vi "Overlay.vi"(9 "RefCnt":cluster{dbl, dbl}[](array[cluster]), 11 "Image In":T1) -> (3 "Image Out":T1)   [LabVIEW 2012]
uses:
  <vilib>/vision/Image Controls.llb/IMAQ Image.ctl
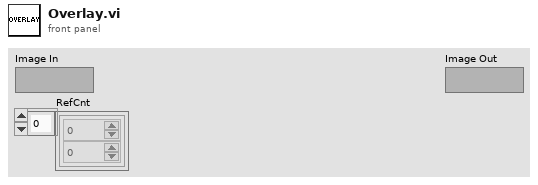
[diagram p1: front panel]
types:
  T1 = typedef "IMAQ Image.ctl" = refnum<image>
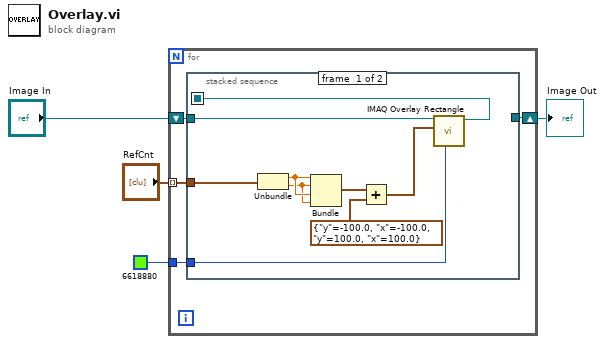
[diagram p0: block diagram]
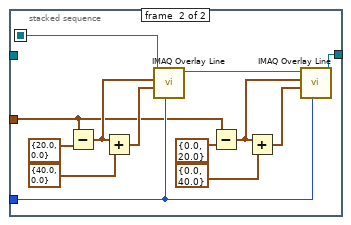
[diagram p2: hidden frame]
diagram:
  n1 = for {
    shift-right: [w7] -> w3
    shift-left: "Image In" -> [w8]
    tunnel: "RefCnt" -> [w6] mode=indexing
    tunnel: u32 6618880 -> [w5]
    n2 = stacked-sequence {
      seq-local: [w16 _] -> [_ w18]
      tunnel: w6 -> [w9 w20]
      tunnel: w8 -> [w17 _]
      tunnel: w5 -> [w15 w22]
      tunnel: [_ w19] -> w7
      frame #0 {
        n3 = Unbundle(w9) -> (w14:dbl, w13:dbl)
        n4 = Bundle(w14, w13, w14, w13) -> (w12:cluster{dbl, dbl, dbl, dbl})  [unwired: 1 out]
        n5 = Add(x=w12, y=cluster{"y":sgl, "x":sgl, "y":sgl, "x":sgl} {"y"=-100.0, "x"=-100.0, "y"=100.0, "x"=100.0}) -> (x+y=w10:cluster{dbl, dbl, dbl, dbl})
        n6 = call "IMAQ Overlay Rectangle"("Color"=w15, "Rectangle"=w10, "Image"=w17) -> ("Image Out"=w16:T1)  [unwired: 7 in, 1 out]
      }
      frame #1 {
        n7 = Subtract(x=w20, y=cluster{"x":sgl, "y":sgl} {"x"=20.0, "y"=0.0}) -> (x-y=w29:cluster{dbl, dbl})
        n8 = Add(x=w29, y=cluster{"x":sgl, "y":sgl} {"x"=40.0, "y"=0.0}) -> (x+y=w27:cluster{dbl, dbl})
        n9 = call "IMAQ Overlay Line"("Color"=w22, "End Point"=w27, "Start Point"=w29, "Image"=w18) -> ("Image Out"=w21:T1)  [unwired: 2 in, 5 out]
        n10 = Subtract(x=w20, y=cluster{"x":sgl, "y":sgl} {"x"=0.0, "y"=20.0}) -> (x-y=w25:cluster{dbl, dbl})
        n11 = Add(x=w25, y=cluster{"x":sgl, "y":sgl} {"x"=0.0, "y"=40.0}) -> (x+y=w26:cluster{dbl, dbl})
        n12 = call "IMAQ Overlay Line"("Color"=w22, "End Point"=w26, "Start Point"=w25, "Image"=w21) -> ("Image Out"=w19:T1)  [unwired: 2 in, 5 out]
      }
    }
  }
  "Image Out" <- w3
